vi "Meas Proc QWTB Update Result View Process.vi"(8 "error in":errorcluster, 11 "session in":variant) -> (0 "error out":errorcluster, 3 "QWTB result session out":variant)   [LabVIEW 2020]
doc: "QWTB result viewer: This VI is async. process that will look into current measurement folder. It scans for results header file, then it reads list of the available results for current QWTB algorithm. It fills the result selector by the list of available results.\nThen it tries to load the result data to the table. It also loads descriptions of the table rows which are stored into the QWTB result session. Alternatively it can generate graph of the selected quantity. The decision table vs graph update is made automatically based on the 'QWTB view setup'."
uses:
  Meas Proc QWTB Plot Legend.ctl
  Meas Proc QWTB Viewer Asyn Session.ctl
  Meas Session.ctl
  adc/ADC Session.ctl
  drivers/niScope/niScope Session.ctl
  drivers/niScope/niScope Virtual Channel Config.ctl
  drivers/niScope/niScope Virtual Channel Mode.ctl
  drivers/niScope/niScope Virtual Channel Input Z.ctl
  drivers/niScope/niScope Virtual Channel Coupling.ctl
  drivers/niScope/niScope Type.ctl
  drivers/niScope/niScope Digitizing Process Options.ctl
  drivers/niScope/niScope Data Packet.ctl
  drivers/niScope/niScope Trigger Setup.ctl
  <instrlib>/niScope/Controls/niScope trigger coupling.ctl
  <instrlib>/niScope/Controls/niScope trigger slope.ctl
  drivers/niScope/niScope Reference Clock.ctl
  drivers/DMM/3458A Digitizer Session.ctl
  drivers/DMM/3458A Virtual Channel Config.ctl
  drivers/Counter/Counter Session.ctl
  drivers/Counter/Counter Type.ctl
  drivers/AWG/AWG Session.ctl
  drivers/AWG/AWG Type.ctl
  drivers/AWG/CMI Clock Divider v2/CMI ckd2 Session.ctl
  drivers/AWG/CMI Clock Divider v2/CMI ckd2 Source Mode.ctl
  drivers/AWG/CMI Clock Divider v2/CMI ckd2 Divisor Mode.ctl
  drivers/AWG/CMI Sync V3/CMI Sync V3 session.ctl
  drivers/AWG/CMI Sync V3/Configure/CMI Sync V3 Reference Clock Source.ctl
  drivers/AWG/CMI Sync V3/Configure/CMI Sync V3 HV input Range.ctl
  drivers/AWG/CMI Sync V3/Configure/CMI Sync V3 Trigger Input Level.ctl
  drivers/AWG/CMI Sync V3/Configure/CMI Sync V3 Channel 1 Mode.ctl
  drivers/AWG/CMI Sync V3/Configure/CMI Sync V3 Channel Output Levels.ctl
  drivers/AWG/CMI Sync V3/Configure/CMI Sync V3 Channel 2 Mode.ctl
  drivers/AWG/CMI Sync V3/Configure/CMI Sync V3 Channel 3 Mode.ctl
  drivers/AWG/CMI Sync V3/Configure/CMI Sync V3 Channel 1 Divisor Entry Mode.ctl
  adc/ADC Trig Config.ctl
  adc/ADC Trig Mode Source.ctl
  adc/ADC Trig Slope.ctl
  adc/ADC Trig Coupling.ctl
  drivers/AWG/RaS HMF2500/HMF2500 Config.ctl
  drivers/DMM/3458A Sync Mode.ctl
  drivers/DMM/3458A Idn Mode.ctl
  drivers/DMM/3458A Digitizing Low Levels/Configure/Sampling Mode.ctl
  drivers/DMM/3458A Digitizing Process Options.ctl
  drivers/DMM/3458A Data Packet.ctl
  drivers/DMM/3458A Aux Record Data.ctl
  drivers/DMM/3458A Digitizing Low Levels/Configure/Level Setup.ctl
  drivers/DMM/3458A Digitizing Low Levels/Configure/First Sample Trigger.ctl
  drivers/DMM/3458A Aperture Selection Mode.ctl
  drivers/DMM/3458A Multiplexing Config.ctl
  drivers/Fluke 8588A/F8588A Low Pass Filter.ctl
  drivers/Fluke 8588A/F8588A Phase Lock.ctl
  drivers/Fluke 8588A/F8588A Coupling.ctl
  drivers/DMM/3458A Sampling Rate.ctl
  drivers/AWG/AWG Clock Setup Mode.ctl
  drivers/DMM/3458A Sample Rate Mode.ctl
  drivers/dsdll/DSDLL Session.ctl
  drivers/dsdll/dsdll/dsdll_instance.ctl
  drivers/dsdll/dsdll/dsdll_device_record.ctl
  drivers/dsdll/DSDLL Process Config.ctl
  drivers/dsdll/DSDLL Data Packet.ctl
  adc/ADC Type.ctl
  drivers/simulated_adc/SimAdc Config.ctl
  drivers/simulated_adc/SimAdc Channel Cfg.ctl
  adc/ADC On Close Action.ctl
  adc/Multiplexer/MPX Session.ctl
  adc/Multiplexer/MPX Type.ctl
  drivers/Multiplexers/Generic COM/GCOMM Session.ctl
  drivers/Multiplexers/Generic COM/GCOMM Signal.ctl
  drivers/Multiplexers/Generic COM/GCOMM Virtual Channel.ctl
  drivers/Multiplexers/Generic COM/GCOMM Logic State.ctl
  drivers/Multiplexers/Generic COM/QPMX Session.ctl
  drivers/Multiplexers/QPMX/QPMX switch mode.ctl
  drivers/Multiplexers/QPMX/QPMX polarity.ctl
  drivers/Multiplexers/Generic VISA commands/GVISA Mux Session.ctl
  drivers/Multiplexers/Generic VISA commands/GVISA Mux Path Entry.ctl
  drivers/Multiplexers/Generic VISA commands/met_serial_setup.ctl
  drivers/Agilent DSO 90000/Virtual Digitizer/KeDSO session.ctl
  drivers/Agilent DSO 90000/Virtual Digitizer/KeDSO Virtual Channel.ctl
  drivers/Agilent DSO 90000/Virtual Digitizer/KeDSO High Resolution Mode.ctl
  drivers/Agilent DSO 90000/Virtual Digitizer/KeDSO Trigger Setup.ctl
  drivers/Agilent DSO 90000/Virtual Digitizer/KeDSO Trigger Source.ctl
  drivers/Agilent DSO 90000/Public/Utility/DSO type.ctl
  drivers/cdaq/cDAQ Session.ctl
  drivers/cdaq/low_level_old/cdaq_anal_adc_command.ctl
  drivers/cdaq/low_level_old/cdaq_anal_adc_data.ctl
  drivers/cdaq/cDAQ Virtual Channel.ctl
  drivers/cdaq/cDAQ Master Clock Mode.ctl
  drivers/CMI_ADS127L21/CMI ADS127L21 - Session.ctl
  drivers/CMI_ADS127L21/CMI ADS127L21 - Record Channel.ctl
  drivers/CMI_ADS127L21/CMI ADS127L21 - Input Range.ctl
  drivers/CMI_ADS127L21/CMI ADS127L21 - Input Mode.ctl
  drivers/CMI_ADS127L21/CMI ADS127L21 - Input Impedance.ctl
  drivers/CMI_ADS127L21/CMI ADS127L21 - EXTOUT Mode.ctl
  drivers/CMI_ADS127L21/CMI ADS127L21 - EXTOUT Polarity.ctl
  Meas Sequence Item.ctl
  Meas Sampling Configuration.ctl
  Meas Proc QWTB Algorithm Parameter Data.ctl
  Meas Sequence Configuration.ctl
  Meas Range Mode.ctl
  Meas Sampling Rate Mode.ctl
  octave/golpi/mpc/golpi_session_ref.ctl
  Meas Process Config.ctl
  Meas Process Mode.ctl
  Meas Process Raw Config.ctl
  Meas Process Raw Result Mode.ctl
  Meas Proc QWTB Setup.ctl
  Meas Proc QWTB Uncertainty Mode.ctl
  Meas Proc QWTB Multicore Setup.ctl
  Meas Proc QWTB Multicore Type.ctl
  Meas Process Time Stamp Mode.ctl
  Meas Proc QWTB Exec Mode.ctl
  Corrections/Corr Setup.ctl
  Corrections/Corr Tranducer Item.ctl
  Corrections/Corr Digitizers.ctl
  Assist/Assist Panel Setup.ctl
  Meas Proc QWTB Viewer References.ctl
  Meas Proc QWTB Update Flags.ctl
  Meas Proc QWTB Plot Config.ctl
  Meas Proc QWTB Plot Scale Mode.ctl
  <vilib>/Utility/miscctls.llb/LVRowAndColumnUnsignedTypeDef.ctl
  varilib/SGUI Assign Multiple Strings With Tags By Label.vi
  octave/infolib/1D String.vi
  octave/infolib/Get 1D String.vi
  octave/golpi/Get String.vi
  octave/golpi/Get Double.vi
  octave/golpi/Get 1D Array Double.vi
  octave/golpi/Get 2D Array Double.vi
  octave/golpi/mpc/GOLPI Multi Process.lvlib
  octave/golpi/GOLPI library.lvlib
  varilib/varilib.lvlib
  drivers/niScope/niScope Virtual Digitizer.lvlib
  drivers/DMM/3458A Virtual Digitizer.lvlib
  drivers/Counter/Counter.lvlib
  drivers/AWG/AWG.lvlib
  drivers/DMM/3458A Digitizing Low Levels/3458A Digitizing Low Levels.lvlib
  drivers/dsdll/DSDLL Virtual Digitizer.lvlib
  octave/infolib/infolib.lvlib
  drivers/dsdll/dsdll/dsdll.lvlib
  drivers/AWG/CMI Sync V3/CMI Sync Unit V3.lvlib
  drivers/Agilent DSO 90000/Agilent 90000 Series.lvlib
panel:
  out "user session (memory)":path
  in  "Show legend":T1
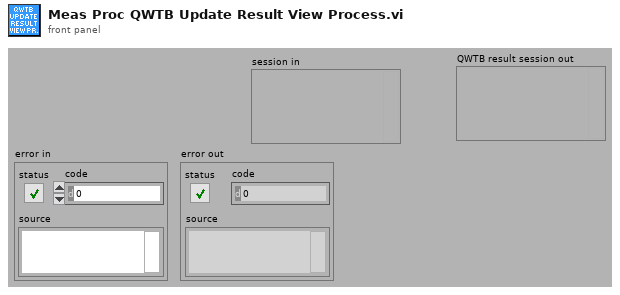
[diagram p1: front panel]
types:
  T1 = typedef "Meas Proc QWTB Plot Legend.ctl" = enum16{"None", "Best", "North", "South", "East", "West", "NorthEast", "NorthWest", "SouthEast", "SouthWest"}
  T2 = typedef "Meas Proc QWTB Viewer Asyn Session.ctl" = cluster{"session":T3, "QWTB result refs":T112, "view setup":T113}
  T3 = typedef "Meas Session.ctl" = cluster{"adc":T4, "sequence":T91[], "sequence setup":T94, "golpi":T97, "processing setup":T98, "corrections":T108, "assist cfg":T111}
  T4 = typedef "ADC Session.ctl" = cluster{"niScope":T5, "3458A":T16, "dsdll":T55, "type":T59, "channel idn str":string[], "aux instr idn str":string[], "modified?":bool, "simadc":T60, "force rst?":bool, "exit mode":T62, "exit dly":dbl, "exit tmr":timestamp, "busy?":bool, "accessed?":bool, "multiplex":T63, "keysight dso":T75, "cdaq":T81, "ignore overload":bool, "ADS127L21":T84}
  T5 = typedef "niScope Virtual Digitizer.lvlib/niScope Session.ctl" = cluster{"channel cfg":T6[], "sessions":refnum<k20>[], "multi cards":bool, "channels":i32, "type":T10, "memory [B/chn]":i32, "ext. clock [Hz]":dbl, "samples count":i64, "use streaming":bool, "proc setup":T11, "sample width [B]":i32, "ranges [V]":dbl[], "trigger setup":T12, "fs [Hz]":dbl, "bitres [bit]":i32, "clock source":T15}
  T6 = typedef "niScope Virtual Digitizer.lvlib/niScope Virtual Channel Config.ctl" = cluster{"Address":refnum<k15>, "Channel":i32, "Mode":T7, "Input Z":T8, "Coupling":T9, "Range [Vpk]":dbl, "btn clr":bool, "btn up":bool, "btn down":bool}
  T7 = typedef "niScope Virtual Digitizer.lvlib/niScope Virtual Channel Mode.ctl" = enum16{"Single ended", "Unbal. differential", "Differential"}
  T8 = typedef "niScope Virtual Digitizer.lvlib/niScope Virtual Channel Input Z.ctl" = enum16{"1 MOhm", "50 Ohm"}
  T9 = typedef "niScope Virtual Digitizer.lvlib/niScope Virtual Channel Coupling.ctl" = enum16{"AC", "DC", "GND"}
  T10 = typedef "niScope Virtual Digitizer.lvlib/niScope Type.ctl" = enum16{"n/a", "5922"}
  T11 = typedef "niScope Virtual Digitizer.lvlib/niScope Digitizing Process Options.ctl" = cluster{"packet size [smpl]":i64, "current timeout [s]":dbl, "blk2blk timeout [s]":dbl, "event time":timestamp, "temp sampl T [s]":dbl, "data queue":refnum<queue>, "stop notifier":refnum<notifier>, "proc ref":refnum<vi>}
  T12 = typedef "niScope Virtual Digitizer.lvlib/niScope Trigger Setup.ctl" = cluster{"coupling":T13, "level [V]":dbl, "slope":T14, "mode":enum16{"Immediate", "External", "Level"}, "pre-trigger [%]":dbl}
  T13 = typedef "niScope trigger coupling.ctl" = u16
  T14 = typedef "niScope trigger slope.ctl" = i32
  T15 = typedef "niScope Virtual Digitizer.lvlib/niScope Reference Clock.ctl" = enum16{"VAL_NO_SOURCE", "VAL_CLK_IN", "VAL_PXI_CLOCK", "VAL_EXTERNAL"}
  T16 = typedef "3458A Virtual Digitizer.lvlib/3458A Digitizer Session.ctl" = cluster{"channels":T17[], "sync unit":T18, "awg unit":T20, "sync mode":T39, "streaming mode":bool, "idn mode":T40, "sampling mode":T41, "sample memory [B]":i32, "proc setup":T42, "sample size [B]":i32, "sample count":i32, "aux data":T44, "ranges [V]":dbl[], "aperture [s]":dbl, "LEVEL trigger":T45, "trigger mode":T46, "measure temp.?":bool, "disp mesages":string[], "shared bus?":bool, "disable display?":bool, "aper mode":T47, "aper rules":dbl[][], "multiplex":T48, "F8588 lpf":T49, "F8588 pll":T50, "F8588 couple":T51, "fs":T52, "fs mode":T54, "init timestamp":timestamp, "last report timestamp":timestamp}
  T17 = typedef "3458A Virtual Digitizer.lvlib/3458A Virtual Channel Config.ctl" = cluster{"VISA":refnum<visa-resource-name>, "Range [Vpk]":dbl, "btn clr":bool, "btn up":bool, "btn down":bool, "F8588":bool, "F8588 guard":bool}
  T18 = typedef "Counter.lvlib/Counter Session.ctl" = cluster{"VISA":refnum<visa-resource-name>, "type":T19}
  T19 = typedef "Counter.lvlib/Counter Type.ctl" = enum16{"Picotest U6200A", "dummy"}
  T20 = typedef "AWG.lvlib/AWG Session.ctl" = cluster{"type":T21, "VISA":refnum<visa-resource-name>, "enable 10MHz ref":bool, "cmi ckd2":T22, "cmi sync v3":T25, "trigger":T34, "HMF2500 cfg":T38}
  T21 = typedef "AWG.lvlib/AWG Type.ctl" = enum16{"Agilent 331xxA to 332xxA", "Agilent 335xxA to 336xxA", "Tektronix AFG3101C", "R&S HMF25xx", "CMI Clock Divider v2", "CMI Sync Unit V3", "dummy"}
  T22 = typedef "AWG.lvlib/CMI ckd2 Session.ctl" = cluster{"VISA":refnum<visa-resource-name>, "clock source":T23, "manual ref clk":bool, "ref clock [Hz]":dbl, "div mode":T24}
  T23 = typedef "AWG.lvlib/CMI ckd2 Source Mode.ctl" = enum16{"Auto", "LF clock", "HF clock", "Internal"}
  T24 = typedef "AWG.lvlib/CMI ckd2 Divisor Mode.ctl" = enum16{"Set divisor directly", "Set divisor by frequency"}
  T25 = typedef "AWG.lvlib/CMI Sync Unit V3.lvlib/CMI Sync V3 session.ctl" = cluster{"VISA":refnum<visa-resource-name>, "baud rate [bd/s]":i32, "source":T26, "hv range":T27, "fsrc is fixed":bool, "fsrc [Hz]":dbl, "freq integ [s]":dbl, "freq filter":i32, "trig level":T28, "chn1 mode":T29, "chn1 level":T30, "chn2 mode":T31, "chn2 level":T30, "chn2 div":i32, "chn3 mode":T32, "chn3 level":T30, "chn1 div entry":T33, "chn1 dev limit [%]":dbl, "chn1 check dev":bool}
  T26 = typedef "AWG.lvlib/CMI Sync Unit V3.lvlib/CMI Sync V3 Reference Clock Source.ctl" = enum16{"Auto", "Internal", "Logic", "Sine", "HV"}
  T27 = typedef "AWG.lvlib/CMI Sync Unit V3.lvlib/CMI Sync V3 HV input Range.ctl" = enum16{"10V", "60V", "250V", "1kV"}
  T28 = typedef "AWG.lvlib/CMI Sync Unit V3.lvlib/CMI Sync V3 Trigger Input Level.ctl" = enum16{"LVCMOS 3V3", "TTL 5V"}
  T29 = typedef "AWG.lvlib/CMI Sync Unit V3.lvlib/CMI Sync V3 Channel 1 Mode.ctl" = enum16{"Source divider", "DDS absolute", "DDS ratio", "DDS ratio M/N"}
  T30 = typedef "AWG.lvlib/CMI Sync Unit V3.lvlib/CMI Sync V3 Channel Output Levels.ctl" = enum16{"Positive 3V3", "Negative 3V3", "Positive 5V", "Negative 5V"}
  T31 = typedef "AWG.lvlib/CMI Sync Unit V3.lvlib/CMI Sync V3 Channel 2 Mode.ctl" = enum16{"Source divider", "Chn 1 divide"}
  T32 = typedef "AWG.lvlib/CMI Sync Unit V3.lvlib/CMI Sync V3 Channel 3 Mode.ctl" = enum16{"Chn 1 Active", "Chn 2 Active", "Chn 1 Trigger", "Chn 2 Trigger", "Gate", "PPS", "10MHz"}
  T33 = typedef "AWG.lvlib/CMI Sync Unit V3.lvlib/CMI Sync V3 Channel 1 Divisor Entry Mode.ctl" = enum16{"Set divisor directly", "Calculate nearest divisor from measured fx"}
  T34 = typedef "ADC Trig Config.ctl" = cluster{"source":T35, "slope":T36, "coupling":T37, "level [V]":dbl, "hysteresis [V]":dbl, "pre-trigger [%]":dbl}
  T35 = typedef "ADC Trig Mode Source.ctl" = enum16{"Immediate", "External", "Level"}
  T36 = typedef "ADC Trig Slope.ctl" = enum16{"POS", "NEG"}
  T37 = typedef "ADC Trig Coupling.ctl" = enum16{"DC", "AC"}
  T38 = typedef "AWG.lvlib/HMF2500 Config.ctl" = cluster{"Baud Rate":u32, "Parity":u16, "Data Bits":u16, "Flow Control":u16}
  T39 = typedef "3458A Virtual Digitizer.lvlib/3458A Sync Mode.ctl" = enum16{"MASTER-SLAVE, MASTER clocked by TIMER", "MASTER-SLAVE, MASTER clocked by AWG", "ALL clocked by AWG", "MASTER-SLAVE, ALL clocked by TIMER", "ALL clocked by AWG with DFLL"}
  T40 = typedef "3458A Virtual Digitizer.lvlib/3458A Idn Mode.ctl" = enum16{"Auto", "Sequential (chn A, chn B, ...)", "From calibration string"}
  T41 = typedef "3458A Virtual Digitizer.lvlib/3458A Digitizing Low Levels.lvlib/Sampling Mode.ctl" = enum16{"DCV", "DSDC", "DSAC"}
  T42 = typedef "3458A Virtual Digitizer.lvlib/3458A Digitizing Process Options.ctl" = cluster{"channel id":i32, "packet size [smpl]":i32, "current timeout [s]":dbl, "blk2blk timeout [s]":dbl, "event time":timestamp, "stop notifier":refnum<notifier>, "data queues":refnum<queue>[], "proc refs":refnum<vi>[], "bus semaphore":T43}
  T43 = typedef "Semaphore RefNum" = refnum<k1>
  T44 = typedef "3458A Virtual Digitizer.lvlib/3458A Aux Record Data.ctl" = cluster{"channel id":i32, "valid?":bool[], "gain [V]":dbl[], "timestamp [s]":dbl[], "Ts [s]":dbl, "abs timestamp":timestamp, "t [deg C]":dbl[], "multiplex timestamp [s]":dbl, "only multiplex?":bool, "multiplex smpl offset":i64, "overflow?":bool}
  T45 = typedef "3458A Virtual Digitizer.lvlib/3458A Digitizing Low Levels.lvlib/Level Setup.ctl" = cluster{"edge":enum16{"POS", "NEG"}, "level [V]":dbl, "coupling":enum16{"DC", "AC"}}
  T46 = typedef "3458A Virtual Digitizer.lvlib/3458A Digitizing Low Levels.lvlib/First Sample Trigger.ctl" = enum16{"AUTO", "EXT", "SYN", "SGL", "HOLD", "LEVEL"}
  T47 = typedef "3458A Virtual Digitizer.lvlib/3458A Aperture Selection Mode.ctl" = enum16{"Manual", "Maximum", "Table"}
  T48 = typedef "3458A Virtual Digitizer.lvlib/3458A Multiplexing Config.ctl" = cluster{"cycles":i32, "delay [s]":dbl, "enabled":bool, "overhead [s]":dbl, "tot smpls":i64, "sub-rec":i32, "overhead [%]":dbl, "emulated":bool}
  T49 = typedef "F8588A Low Pass Filter.ctl" = enum16{"Off", "100 kHz", "3 MHz"}
  T50 = typedef "F8588A Phase Lock.ctl" = enum16{"Off", "1 MHz", "10 MHz"}
  T51 = typedef "F8588A Coupling.ctl" = enum16{"AC, 1 MOhm", "AC, 10 MOhm", "DC, 1 MOhm", "DC, 10 MOhm", "DC, auto"}
  T52 = typedef "3458A Virtual Digitizer.lvlib/3458A Sampling Rate.ctl" = cluster{"freq mode":T53, "fs [Hz]":dbl, "fref [Hz]":dbl, "mul":dbl, "div":dbl}
  T53 = typedef "AWG.lvlib/AWG Clock Setup Mode.ctl" = enum16{"fs or Ts", "fs or Ts with fref", "fref/N", "fref*M/N", "fref*Ratio"}
  T54 = typedef "3458A Sample Rate Mode.ctl" = enum16{"fs or Ts", "fs*M/N"}
  T55 = typedef "DSDLL Virtual Digitizer.lvlib/DSDLL Session.ctl" = cluster{"dsdll":T56, "channels":i32, "device id":i32, "channel idns":string[], "proc setup":T58, "samples count":i32, "fs [Hz]":dbl}
  T56 = typedef "dsdll.lvlib/dsdll_instance.ctl" = cluster{"dsdll path":path, "dsdll handle":u8[], "output devices":T57[], "capture devices":T57[]}
  T57 = typedef "dsdll.lvlib/dsdll_device_record.ctl" = cluster{"guid":u8[], "name":string}
  T58 = typedef "DSDLL Virtual Digitizer.lvlib/DSDLL Process Config.ctl" = cluster{"packet size [smpl]":i32, "current timeout [s]":dbl, "blk2blk timeout [s]":dbl, "event time":timestamp, "data queue":refnum<queue>, "stop notifier":refnum<notifier>, "proc ref":refnum<vi>}
  T59 = typedef "ADC Type.ctl" = enum16{"niScope", "3458A", "DirectSound DLL", "Keysight DSO", "cDAQ ADC", "CMI ADS127L21", "dummy"}
  T60 = typedef "SimAdc Config.ctl" = cluster{"channels":T61[], "range [V]":dbl, "Ts step [s]":dbl, "time [s]":dbl, "fs [Hz]":dbl, "count":i64, "smpl offset":i64, "set count":i64, "bit res":i32}
  T61 = typedef "SimAdc Channel Cfg.ctl" = cluster{"harmonics":dbl[][], "btn clear":bool, "noise":dbl, "fundamental [Hz]":dbl}
  T62 = typedef "ADC On Close Action.ctl" = enum16{"Immediate reset", "Delayed reset"}
  T63 = typedef "MPX Session.ctl" = cluster{"Type":T64, "gen com ssn":T65, "delay before [s]":dbl, "delay post [s]":dbl, "sequence":string[], "enabled":bool, "ref timestamp [s]":dbl, "idn string":string, "dev niScope":refnum<k15>, "niScope idx":i32, "QPMX ssn":T69, "VISA mux ssn":T72}
  T64 = typedef "MPX Type.ctl" = enum16{"Dummy", "Generic - COM port", "Generic - niScope PFI", "Generic - VISA commands", "QPMX"}
  T65 = typedef "GCOMM Session.ctl" = cluster{"visa":refnum<visa-resource-name>, "primary":T66, "secondary":T66, "channels":T67[]}
  T66 = typedef "GCOMM Signal.ctl" = enum16{"None", "DTR", "RTS"}
  T67 = typedef "GCOMM Virtual Channel.ctl" = cluster{"Primary:":T68, "Secondary:":T68, "btn clr":bool, "btn up":bool, "btn down":bool, "Tag:":string}
  T68 = typedef "GCOMM Logic State.ctl" = enum16{"OFF", "ON"}
  T69 = typedef "QPMX Session.ctl" = cluster{"visa":refnum<visa-resource-name>, "switch mode":T70, "sequence":bool[][], "timing delays":u32[], "polarity":T71, "ss delay (s)":dbl, "internal timer (s)":dbl, "Last loaded sequence file":path, "startup delay (s)":dbl}
  T70 = typedef "QPMX switch mode.ctl" = enum16{"Switched by TWM", "Switched by external clock", "Switched by internal clock"}
  T71 = typedef "QPMX polarity.ctl" = enum16{"Positive", "Negative"}
  T72 = typedef "GVISA Mux Session.ctl" = cluster{"VISA":refnum<visa-resource-name>, "paths":T73[], "idn command":string, "serial cfg":T74}
  T73 = typedef "GVISA Mux Path Entry.ctl" = cluster{"Tag:":string, "Command:":string, "btn clr":bool, "btn up":bool, "btn down":bool}
  T74 = typedef "met_serial_setup.ctl" = cluster{"Baud rate":i32, "Data bits":i32, "Parity":i32, "Stop bits":i32, "Flow control":i32, "End Mode Read":enum16{"None", "Last Bit", "TermChar"}, "End Mode Write":enum16{"None", "Last Bit", "TermChar"}, "Term character":u8, "Term enable":bool}
  T75 = typedef "KeDSO session.ctl" = cluster{"VISA":refnum<visa-resource-name>, "channels":T76[], "bw limit [Hz]":dbl, "resolution":T77, "trig noise reject":enum16{"Normal", "High Sensitivity"}, "N":i64, "trigger config":T78, "fs [Hz]":dbl, "timeout stop":timestamp, "waiting for opc":bool, "fetch offset [smpl]":i64, "abs timestamp":timestamp, "ranges [V]":dbl[], "decimation":dbl, "ext ref":bool, "emulate aperture":bool, "model":T80}
  T76 = typedef "KeDSO Virtual Channel.ctl" = cluster{"Channel":i32, "Range [Vpk]":dbl, "btn clr":bool, "btn up":bool, "btn down":bool, "Offset [V]":dbl, "Coupling":enum16{"DC", "DC50", "AC", "LFR1"}, "bw limit enab":bool}
  T77 = typedef "KeDSO High Resolution Mode.ctl" = enum16{"Basic", "High-res AUTO", "Min. 9-bits", "Min. 10-bits", "Min. 11-bits", "Min. 12-bits", "Fixed 11-bits", "Fixed 12-bits", "Fixed 13-bits", "Fixed 14-bits", "Fixed 15-bits", "Fixed 16-bits"}
  T78 = typedef "KeDSO Trigger Setup.ctl" = cluster{"trigger source":T79, "trigger slope":enum16{"Negative", "Positive", "Either"}, "level [V]":dbl, "hysteresis [V]":dbl, "pre-trig [%]":i32}
  T79 = typedef "KeDSO Trigger Source.ctl" = enum16{"Immediate", "Level", "AUX"}
  T80 = typedef "Agilent 90000 Series.lvlib/DSO type.ctl" = enum16{"DSO91304", "DSO91204", "DSO90804", "DSO90604", "DSO90404", "DSO90254", "DSA91304", "DSA91204", "DSA90804", "DSA90604", "DSA90404", "DSA90254", "DSO9104", "DSO9254", "DSO9404", "MSO9104", "MSO9254", "MSO9404", "MSO9064", "DSO9064", "DSOX91604", "DSOX92004", "DSOX92504", "DSOX92804", "DSOX93204", "DSO93004", "DSO9024H", "DSO9054H", "DSO9104H", "DSO9204H", "DSOS054A", "DSOS104A", "DSOS204A", "DSOS254A", "DSOS404A", "DSOS604A", "DSOS804A", "MSOS054A", "MSOS104A", "MSOS204A", "MSOS254A", "MSOS404A", "MSOS604A", "MSOS804A", "DSAX96204Q", "DSOX96204Q", "DSAX95004Q", "DSOX95004Q", "DSAX93304Q", "DSOX93304Q", "DSAX92504Q", "DSOX92504Q", "DSAX92004Q", "DSOX92004Q"}
  T81 = typedef "cDAQ Session.ctl" = cluster{"mclk [Hz]":dbl, "ADC task":refnum<k21>, "mclk reference":string, "fs [Hz]":dbl, "queue adc cmd":refnum<queue>, "queue adc data":refnum<queue>, "adc proc ref":refnum<vi>, "channels":T82[], "last channels":T82[], "timeout":timestamp, "N":i32, "mclk mode":T83, "ext mclk source":tag}
  T82 = typedef "cDAQ Virtual Channel.ctl" = cluster{"Device":tag, "Channel id":i32, "btn clr":bool, "btn up":bool, "btn down":bool}
  T83 = typedef "cDAQ Master Clock Mode.ctl" = enum16{"Free running", "Export master clock", "Import master clock"}
  T84 = typedef "CMI ADS127L21 - Session.ctl" = cluster{"VISA":refnum<visa-resource-name>, "chn list":i32[], "record size":i32, "phys. channels":i32, "adc fifo size":i32, "channels":T85[], "ext refclk?":bool, "fs [Hz]":dbl, "ext refclk [Hz]":dbl, "meas refclk [Hz]":dbl, "EXTOUT mode":T89, "EXTOUT polarity":T90, "EXTOUT divisor":i32}
  T85 = typedef "CMI ADS127L21 - Record Channel.ctl" = cluster{"Range [Vpk]":T86, "Channel":i32, "Mode":T87, "Impedance":T88, "btn clr":bool, "btn up":bool, "btn down":bool}
  T86 = typedef "CMI ADS127L21 - Input Range.ctl" = dbl
  T87 = typedef "CMI ADS127L21 - Input Mode.ctl" = enum16{"Normal", "Inverted", "GND"}
  T88 = typedef "CMI ADS127L21 - Input Impedance.ctl" = enum16{"1M", "1k5"}
  T89 = typedef "CMI ADS127L21 - EXTOUT Mode.ctl" = enum16{"ADCCLK", "REFCLK", "SMPLCLK", "FIRST"}
  T90 = typedef "CMI ADS127L21 - EXTOUT Polarity.ctl" = enum16{"NORM", "INV"}
  T91 = typedef "Meas Sequence Item.ctl" = cluster{"config":T92, "data file path":path, "header file path":path, "group id":i32, "rec id":i32, "group done?":bool, "adc modified?":bool, "source modified?":bool, "progress [%]":dbl, "groups cnt":i32, "rec cnt":i32, "data file relative path":string, "meas root path":path, "calculate?":bool, "comment":string, "avg cnt":i32}
  T92 = typedef "Meas Sampling Configuration.ctl" = cluster{"count [smpl]":i64, "aperture [s]":dbl, "trigger":T34, "ranges [Vpk]":dbl[], "QWTB parameters":T93[], "sampling rate":T52}
  T93 = typedef "Meas Proc QWTB Algorithm Parameter Data.ctl" = cluster{"name":string, "numerics":dbl[], "strings":string[]}
  T94 = typedef "Meas Sequence Configuration.ctl" = cluster{"group setups":T92[], "rec count":i32, "range mode":T95, "fs mode":T96, "rng even":dbl, "rng odd":dbl, "folder":path, "name base":string, "meas id":i32, "settle [s]":dbl, "comment":string, "avg count":i32, "fs-abs-fr fr":dbl, "fs-abs-fr fs":dbl, "fs-div fr":dbl, "fs-div div":dbl, "fs-mn fr":dbl, "fs-mn mul":dbl, "fs-mn div":dbl, "fs-rat fr":dbl, "fs-rat rat":dbl}
  T95 = typedef "Meas Range Mode.ctl" = enum16{"Keep defaults", "Set All channels", "Set Odd and Even channels"}
  T96 = typedef "Meas Sampling Rate Mode.ctl" = enum16{"Frequency", "Period"}
  T97 = typedef "GOLPI Multi Process.lvlib/golpi_session_ref.ctl" = refnum<vi>
  T98 = typedef "Meas Process Config.ctl" = cluster{"mode":T99, "call after avgs?":bool, "calculate?":bool, "raw mode":T100, "QWTB":T102}
  T99 = typedef "Meas Process Mode.ctl" = enum16{"Raw", "QWTB"}
  T100 = typedef "Meas Process Raw Config.ctl" = cluster{"command":string, "result mode":T101, "res variable":string}
  T101 = typedef "Meas Process Raw Result Mode.ctl" = enum16{"Display console output (only Octave)", "Display string variable", "Display result file %respath%"}
  T102 = typedef "Meas Proc QWTB Setup.ctl" = cluster{"QWTB path":path, "alg filter path":string, "alg ids":string[], "alg parameters":string[], "parsed parameters":T93[], "selected alg id":string, "selected unc mode":T103, "qwtb mcc":i32, "qwtb timeout":i32, "qwtb covg":dbl, "qwtb ofs":i64, "qwtb lim data":i64, "multicore":T104, "unc once?":bool, "qwtb tstemp":T106, "octave reset":bool, "exec mode":T107}
  T103 = typedef "Meas Proc QWTB Uncertainty Mode.ctl" = enum16{"None", "GUF", "Monte Carlo"}
  T104 = typedef "Meas Proc QWTB Multicore Setup.ctl" = cluster{"jobs folder":path, "cores":i32, "max jobs":i32, "mode":T105}
  T105 = typedef "Meas Proc QWTB Multicore Type.ctl" = enum16{"Singlecore", "Multicore", "Multistation"}
  T106 = typedef "Meas Process Time Stamp Mode.ctl" = enum16{"Enabled (default)", "Disabled", "Relative to 1. record"}
  T107 = typedef "Meas Proc QWTB Exec Mode.ctl" = enum16{"Single-core", "Parallel Record Processing"}
  T108 = typedef "Corr Setup.ctl" = cluster{"transducers":cluster{"channels":T109[], "last path":path, "root path":path}, "digitizer":T110}
  T109 = typedef "Corr Tranducer Item.ctl" = cluster{"Path":path, "Ratio:":string, "Name:":string, "btn rem":bool, "btn up":bool, "btn down":bool, "s.n.:":string, "btn open":bool, "ratio o/i":dbl, "chn hi":u16, "chn lo":u16, "Phase index":i32, "btn edit":bool, "mpx chn":u16, "btn vdx1":bool, "btn csx1":bool, "invert":bool}
  T110 = typedef "Corr Digitizers.ctl" = cluster{"last path":path, "channel paths":path[], "channel idns":string[], "correction name":string, "channel names":string[], "folders to copy":path[], "channel valid":bool[], "correction path":path, "correction rel path":string, "rel folders to copy":string[], "root path":path}
  T111 = typedef "Assist Panel Setup.ctl" = cluster{"P":i32, "Q":i32, "rel shift":dbl, "ref freq":dbl, "min fs":dbl, "max fs tol":dbl, "min int":dbl, "max int":dbl, "max err":dbl, "max timeout":dbl}
  T112 = typedef "Meas Proc QWTB Viewer References.ctl" = cluster{"tc result":refnum<vi>, "qwtb results tbl":refnum<vi>, "qwtb maxdim":refnum<vi>, "qwtb unc":refnum<vi>, "qwtb order":refnum<vi>, "qwtb maxarr":refnum<vi>, "qwtb res sel":refnum<vi>, "qwtb res info":refnum<vi>, "descriptions":string[], "var names":string[], "channel indexes":i32[], "qwtb ref chn":refnum<vi>, "qwtb ph unit":refnum<vi>, "qwtb alg sel":refnum<vi>, "qwtb meas sel":refnum<vi>, "qwtb ssn info":refnum<vi>, "last session (man)":path, "qwtb qu list":refnum<vi>, "matrix":dbl[][], "comment":string, "qwtb comment":refnum<vi>, "last session":path, "qwtb amp":refnum<vi>}
  T113 = typedef "Meas Proc QWTB Update Flags.ctl" = cluster{"new result":bool, "show graph":bool, "plot setup":T114, "new session":bool, "reset viewer":bool, "store comment":bool}
  T114 = typedef "Meas Proc QWTB Plot Config.ctl" = cluster{"X-axis style":T115, "Y-axis style":T115, "Show legend":T1, "Grid on":bool, "Box on":bool, "show all chn":bool, "keep updating":bool}
  T115 = typedef "Meas Proc QWTB Plot Scale Mode.ctl" = enum16{"Linear", "Log"}
  T116 = typedef "LVRowAndColumnUnsignedTypeDef.ctl" = cluster{"Row":u32, "Column":u32}
  T117 = typedef "GOLPI library.lvlib/GOLPI reference Type Def.ctl" = cluster{"pipe handle":T118, "fast read timeout [ms]":u32, "fast read settle time [ms]":u32, "fast read to multiple [ms]":u32, "max elements per input line":u32, "slow read timeout [ms]":u32, "stdin double format specifier":string, "max elements per stdout output column":u32, "console mode bitstream":bool, "bitstream first read timeout [ms]":u32, "bitstream read timeout [ms]":u32, "struct transfer possible":bool, "matlab mode":bool}
  T118 = typedef "LV Process library.lvlib/Pipe Handle.ctl" = cluster{"lv_proc.dll file path":path, "process instance handle":u32[], "debug mode":bool, "debug data":cluster{"time":timestamp, "stdin":bool, "data":string}[]}
  T119 = typedef "Meas Proc QWTB View Amplitude Mode.ctl" = enum16{"Amplitude", "Effective", "amp. * sqrt(3)", "amp. / sqrt(3)", "eff. * sqrt(3)", "eff. / sqrt(3)", "Peak-Peak", "dB", "dBmV (dBmA)", "dBuV (dBuA)"}
  T120 = typedef "Meas Proc QWTB View Max Dim.ctl" = enum16{"Scalar", "Vector", "Matrix"}
  T121 = typedef "Meas Proc QWTB View Group Mode.ctl" = enum16{"Group quantities", "Group phases"}
  T122 = typedef "Meas Proc QWTB View Uncertainty Mode.ctl" = enum16{"None", "val ± unc", "[val; unc]"}
  T123 = typedef "Meas Proc QWTB View Phase Mode.ctl" = enum16{"± pi [rad]", "0 - 2*pi [rad]", "±180 [deg]", "0 - 360 [deg]"}
  T124 = typedef "LVRowAndColumnTypeDef.ctl" = cluster{"Row":i32, "Column":i32}
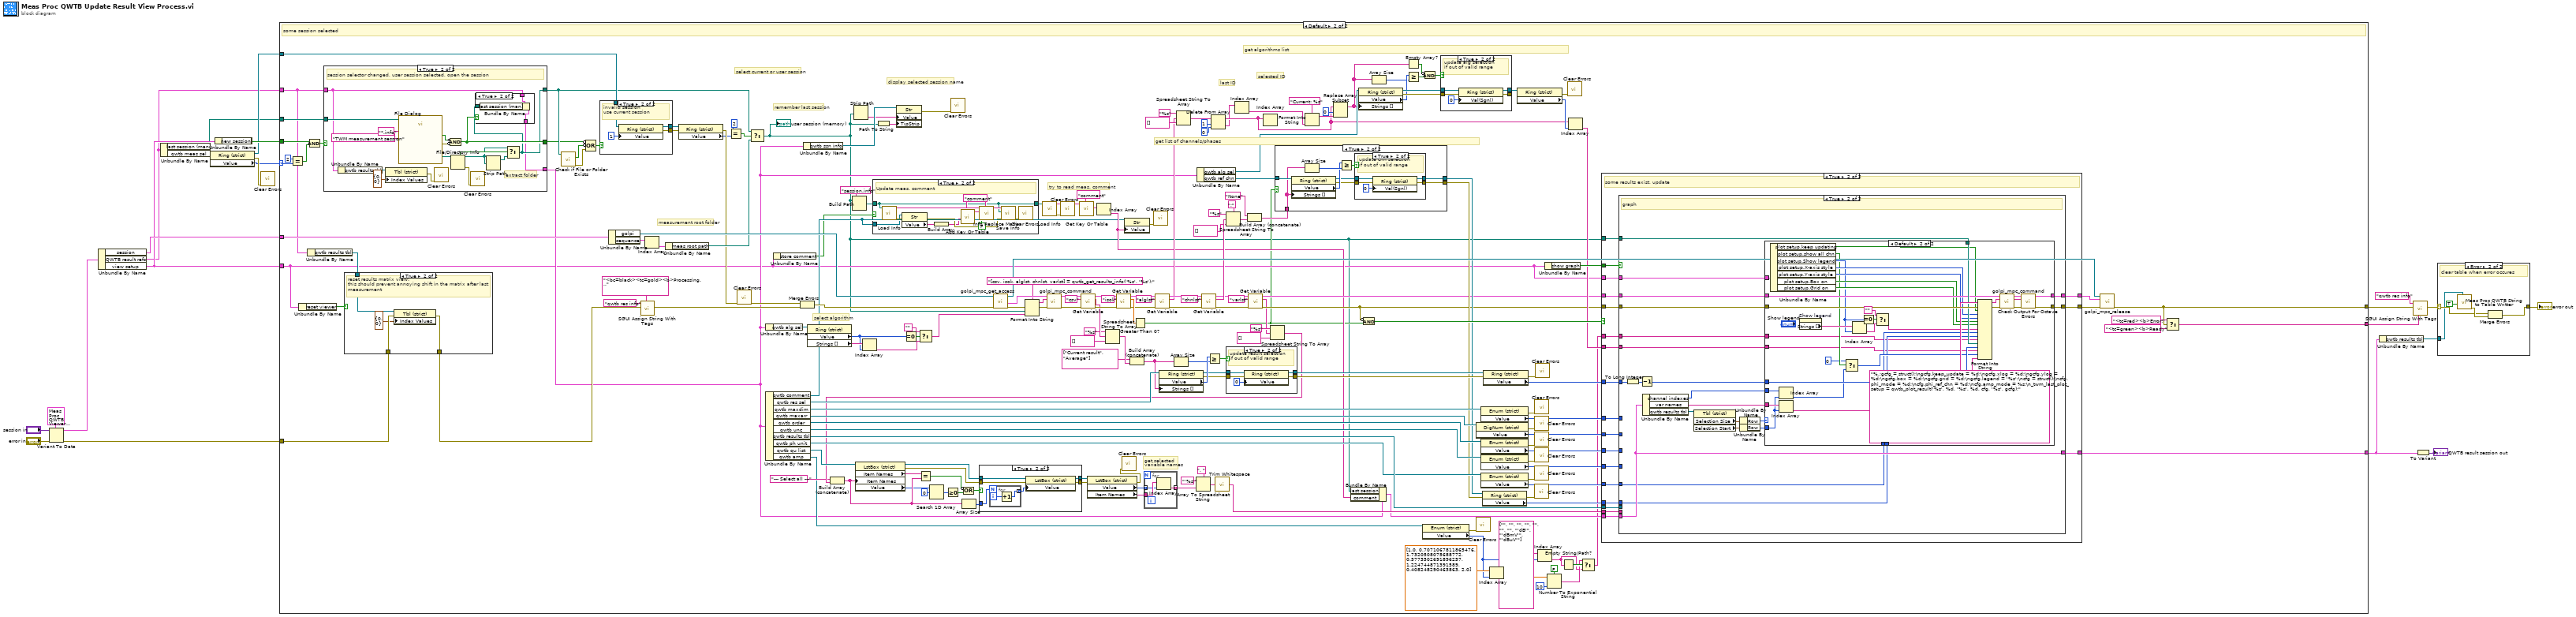
[diagram p0: block diagram]
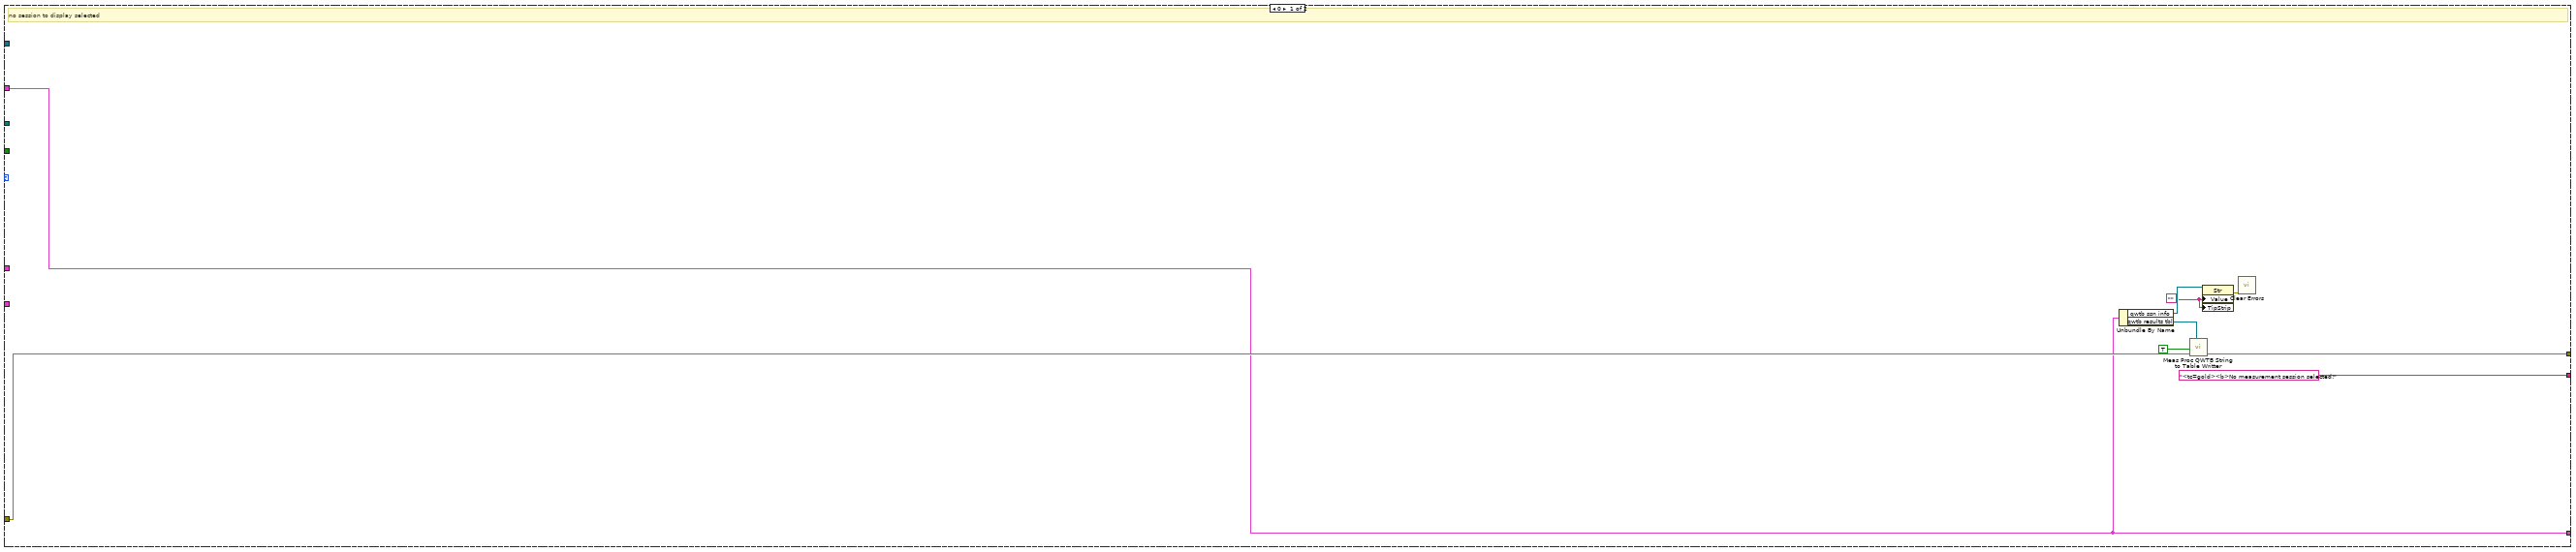
[diagram p3: hidden frame]
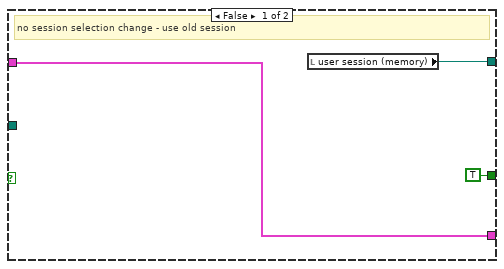
[diagram p10: hidden frame]
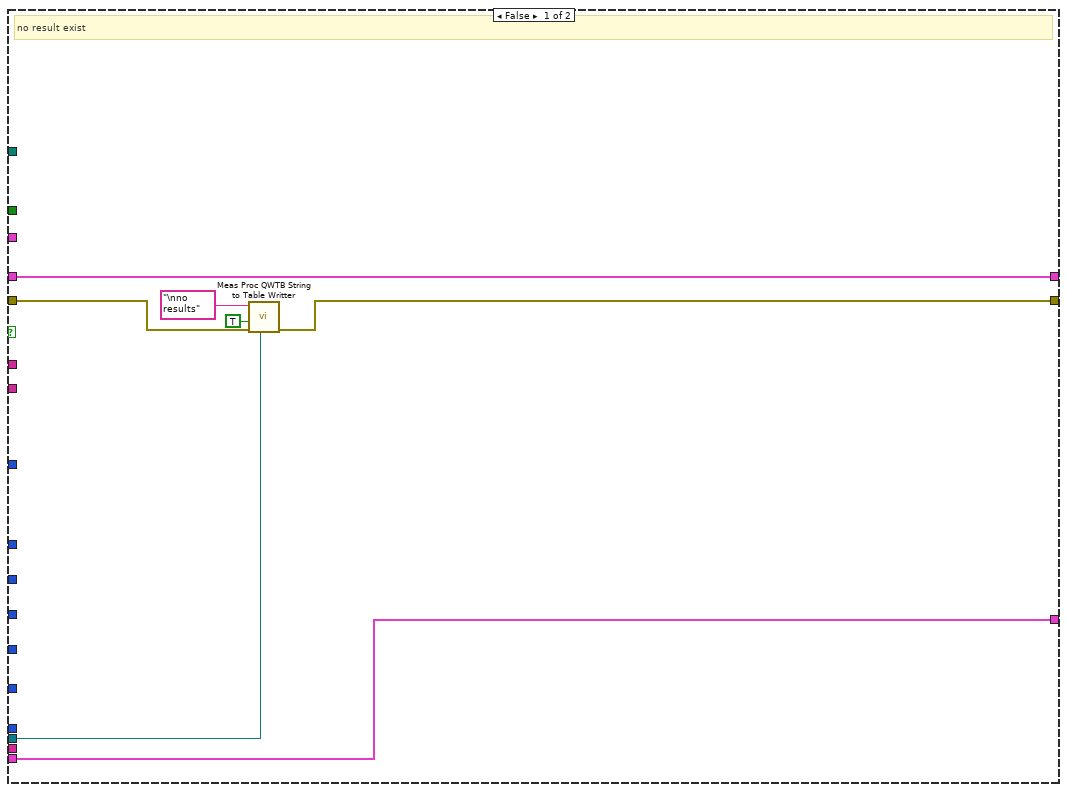
[diagram p13: hidden frame]
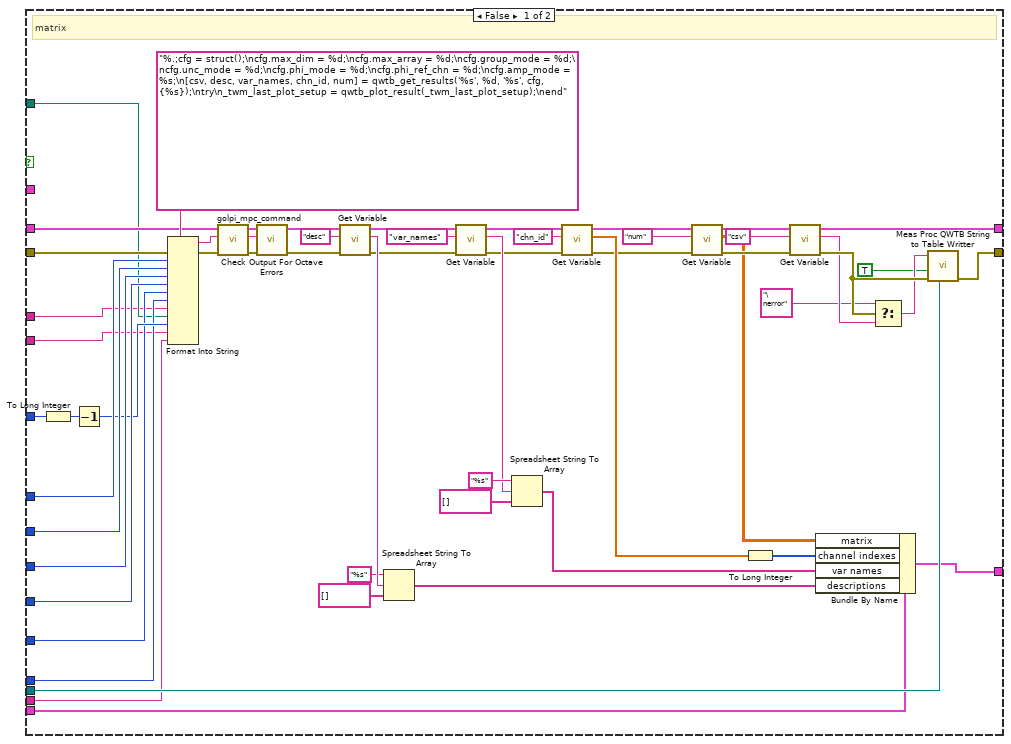
[diagram p14: hidden frame]
diagram:
  n1 = Variant To Data(error in="error in", type=T2 {"session"={"adc"={"niScope"={"channel cfg"=[], "sessions"=[], "multi cards"=FALSE, "channels"=0, "type"=enum."n/a", "memory [B/chn]"=0, "ext. clock [Hz]"=0.0, "samples count"=0, "use streaming"=FALSE, "proc setup"={"packet size [smpl]"=0, "current timeout [s]"=0.0, "blk2blk timeout [s]"=0.0, "event time"=timestamp(0 s since 1904-01-01), "temp sampl T [s]"=0.0, "data queue"=refnum, "stop notifier"=refnum, "proc ref"=refnum}, "sample width [B]"=0, "ranges [V]"=[], "trigger setup"={"coupling"=1, "level [V]"=0.0, "slope"=0, "mode"=enum."Immediate", "pre-trigger [%]"=0.0}, "fs [Hz]"=0.0, "bitres [bit]"=0, "clock source"=enum."VAL_NO_SOURCE"}, "3458A"={"channels"=[], "sync unit"={"VISA"="", "type"=enum."Picotest U6200A"}, "awg unit"={"type"=enum."Agilent 331xxA to 332xxA", "VISA"="", "enable 10MHz ref"=FALSE, "cmi ckd2"={"VISA"="", "clock source"=enum."Auto", "manual ref clk"=FALSE, "ref clock [Hz]"=0.0, "div mode"=enum."Set divisor directly"}, "cmi sync v3"={"VISA"="", "baud rate [bd/s]"=115200, "source"=enum."Auto", "hv range"=enum."1kV", "fsrc is fixed"=FALSE, "fsrc [Hz]"=10000000.0, "freq integ [s]"=1.0, "freq filter"=5, "trig level"=enum."TTL 5V", "chn1 mode"=enum."Source divider", "chn1 level"=enum."Positive 5V", "chn2 mode"=enum."Source divider", "chn2 level"=enum."Positive 5V", "chn2 div"=1, "chn3 mode"=enum."Chn 1 Active", "chn3 level"=enum."Positive 5V", "chn1 div entry"=enum."Calculate nearest divisor from measured fx", "chn1 dev limit [%]"=1.0, "chn1 check dev"=FALSE}, "trigger"={"source"=enum."Immediate", "slope"=enum."POS", "coupling"=enum."DC", "level [V]"=0.0, "hysteresis [V]"=0.0, "pre-trigger [%]"=0.0}, "HMF2500 cfg"={"Baud Rate"=9600, "Parity"=0, "Data Bits"=8, "Flow Control"=4}}, "sync mode"=enum."MASTER-SLAVE, MASTER clocked by TIMER", "streaming mode"=FALSE, "idn mode"=enum."Auto", "sampling mode"=enum."DCV", "sample memory [B]"=0, "proc setup"={"channel id"=0, "packet size [smpl]"=0, "current timeout [s]"=0.0, "blk2blk timeout [s]"=0.0, "event time"=timestamp(0 s since 1904-01-01), "stop notifier"=refnum, "data queues"=[], "proc refs"=[], "bus semaphore"=refnum}, "sample size [B]"=0, "sample count"=0, "aux data"={"channel id"=0, "valid?"=[], "gain [V]"=[], "timestamp [s]"=[], "Ts [s]"=0.0, "abs timestamp"=timestamp(0 s since 1904-01-01), "t [deg C]"=[], "multiplex timestamp [s]"=-1.0, "only multiplex?"=FALSE, "multiplex smpl offset"=0, "overflow?"=FALSE}, "ranges [V]"=[], "aperture [s]"=0.0, "LEVEL trigger"={"edge"=enum."POS", "level [V]"=0.0, "coupling"=enum."DC"}, "trigger mode"=enum."AUTO", "measure temp.?"=FALSE, "disp mesages"=[], "shared bus?"=FALSE, "disable display?"=FALSE, "aper mode"=enum."Manual", "aper rules"=[], "multiplex"={"cycles"=0, "delay [s]"=0.0, "enabled"=FALSE, "overhead [s]"=1.0, "tot smpls"=0, "sub-rec"=0, "overhead [%]"=0.0, "emulated"=FALSE}, "F8588 lpf"=enum."Off", "F8588 pll"=enum."Off", "F8588 couple"=enum."DC, auto", "fs"={"freq mode"=enum."fs or Ts", "fs [Hz]"=0.0, "fref [Hz]"=0.0, "mul"=0.0, "div"=0.0}, "fs mode"=enum."fs or Ts", "init timestamp"=timestamp(0 s since 1904-01-01), "last report timestamp"=timestamp(0 s since 1904-01-01)}, "dsdll"={"dsdll"={"dsdll path"=path "", "dsdll handle"=[], "output devices"=[], "capture devices"=[]}, "channels"=0, "device id"=0, "channel idns"=[], "proc setup"={"packet size [smpl]"=0, "current timeout [s]"=0.0, "blk2blk timeout [s]"=0.0, "event time"=timestamp(0 s since 1904-01-01), "data queue"=refnum, "stop notifier"=refnum, "proc ref"=refnum}, "samples count"=0, "fs [Hz]"=0.0}, "type"=enum."niScope", "channel idn str"=[], "aux instr idn str"=[], "modified?"=FALSE, "simadc"={"channels"=[], "range [V]"=0.0, "Ts step [s]"=0.0, "time [s]"=0.0, "fs [Hz]"=0.0, "count"=0, "smpl offset"=0, "set count"=0, "bit res"=0}, "force rst?"=FALSE, "exit mode"=enum."Immediate reset", "exit dly"=0.0, "exit tmr"=timestamp(0 s since 1904-01-01), "busy?"=FALSE, "accessed?"=FALSE, "multiplex"={"Type"=enum."Dummy", "gen com ssn"={"visa"="", "primary"=enum."None", "secondary"=enum."None", "channels"=[]}, "delay before [s]"=0.0, "delay post [s]"=0.0, "sequence"=[], "enabled"=FALSE, "ref timestamp [s]"=0.0, "idn string"="", "dev niScope"="", "niScope idx"=0, "QPMX ssn"={"visa"="", "switch mode"=enum."Switched by TWM", "sequence"=[], "timing delays"=[], "polarity"=enum."Positive", "ss delay (s)"=2.0, "internal timer (s)"=1.0, "Last loaded sequence file"=path "", "startup delay (s)"=2.0}, "VISA mux ssn"={"VISA"="", "paths"=[], "idn command"="", "serial cfg"={"Baud rate"=9600, "Data bits"=8, "Parity"=0, "Stop bits"=10, "Flow control"=0, "End Mode Read"=enum."None", "End Mode Write"=enum."None", "Term character"=0, "Term enable"=FALSE}}}, "keysight dso"={"VISA"="", "channels"=[], "bw limit [Hz]"=0.0, "resolution"=enum."Basic", "trig noise reject"=enum."Normal", "N"=0, "trigger config"={"trigger source"=enum."Immediate", "trigger slope"=enum."Negative", "level [V]"=0.0, "hysteresis [V]"=0.001, "pre-trig [%]"=50}, "fs [Hz]"=0.0, "timeout stop"=timestamp(0 s since 1904-01-01), "waiting for opc"=FALSE, "fetch offset [smpl]"=0, "abs timestamp"=timestamp(0 s since 1904-01-01), "ranges [V]"=[], "decimation"=1.0, "ext ref"=FALSE, "emulate aperture"=FALSE, "model"=enum."DSO91304"}, "cdaq"={"mclk [Hz]"=12800000.0, "ADC task"="", "mclk reference"="", "fs [Hz]"=50000.0, "queue adc cmd"=refnum, "queue adc data"=refnum, "adc proc ref"=refnum, "channels"=[], "last channels"=[], "timeout"=timestamp(0 s since 1904-01-01), "N"=1000, "mclk mode"=enum."Free running", "ext mclk source"=""}, "ignore overload"=FALSE, "ADS127L21"={"VISA"="", "chn list"=[], "record size"=0, "phys. channels"=0, "adc fifo size"=0, "channels"=[], "ext refclk?"=FALSE, "fs [Hz]"=0.0, "ext refclk [Hz]"=0.0, "meas refclk [Hz]"=0.0, "EXTOUT mode"=enum."ADCCLK", "EXTOUT polarity"=enum."NORM", "EXTOUT divisor"=0}}, "sequence"=[], "sequence setup"={"group setups"=[], "rec count"=0, "range mode"=enum."Keep defaults", "fs mode"=enum."Frequency", "rng even"=0.0, "rng odd"=0.0, "folder"=path "", "name base"="", "meas id"=0, "settle [s]"=0.0, "comment"="", "avg count"=0, "fs-abs-fr fr"=0.0, "fs-abs-fr fs"=0.0, "fs-div fr"=0.0, "fs-div div"=0.0, "fs-mn fr"=0.0, "fs-mn mul"=0.0, "fs-mn div"=0.0, "fs-rat fr"=0.0, "fs-rat rat"=0.0}, "golpi"=refnum, "processing setup"={"mode"=enum."Raw", "call after avgs?"=FALSE, "calculate?"=FALSE, "raw mode"={"command"="", "result mode"=enum."Display console output (only Octave)", "res variable"=""}, "QWTB"={"QWTB path"=path "", "alg filter path"="", "alg ids"=[], "alg parameters"=[], "parsed parameters"=[], "selected alg id"="", "selected unc mode"=enum."None", "qwtb mcc"=100, "qwtb timeout"=90, "qwtb covg"=95.0, "qwtb ofs"=0, "qwtb lim data"=0, "multicore"={"jobs folder"=path "", "cores"=0, "max jobs"=0, "mode"=enum."Singlecore"}, "unc once?"=FALSE, "qwtb tstemp"=enum."Enabled (default)", "octave reset"=FALSE, "exec mode"=enum."Single-core"}}, "corrections"={"transducers"={"channels"=[], "last path"=path "", "root path"=path ""}, "digitizer"={"last path"=path "", "channel paths"=[], "channel idns"=[], "correction name"="", "channel names"=[], "folders to copy"=[], "channel valid"=[], "correction path"=path "", "correction rel path"="", "rel folders to copy"=[], "root path"=path ""}}, "assist cfg"={"P"=0, "Q"=0, "rel shift"=0.0, "ref freq"=0.0, "min fs"=0.0, "max fs tol"=0.0, "min int"=0.0, "max int"=0.0, "max err"=0.0, "max timeout"=0.0}}, "QWTB result refs"={"tc result"=refnum, "qwtb results tbl"=refnum, "qwtb maxdim"=refnum, "qwtb unc"=refnum, "qwtb order"=refnum, "qwtb maxarr"=refnum, "qwtb res sel"=refnum, "qwtb res info"=refnum, "descriptions"=[], "var names"=[], "channel indexes"=[], "qwtb ref chn"=refnum, "qwtb ph unit"=refnum, "qwtb alg sel"=refnum, "qwtb meas sel"=refnum, "qwtb ssn info"=refnum, "last session (man)"=path "", "qwtb qu list"=refnum, "matrix"=[], "comment"="", "qwtb comment"=refnum, "last session"=path "", "qwtb amp"=refnum}, "view setup"={"new result"=FALSE, "show graph"=FALSE, "plot setup"={"X-axis style"=enum."Linear", "Y-axis style"=enum."Linear", "Show legend"=enum."None", "Grid on"=FALSE, "Box on"=FALSE, "show all chn"=FALSE, "keep updating"=FALSE}, "new session"=FALSE, "reset viewer"=FALSE, "store comment"=FALSE}} ("Cluster"), Variant="session in") -> (data=w18:T2, error out=w16:errorcluster)
  n2 = Unbundle By Name(w18) -> ("session"=w17:T3, "QWTB result refs"=w9:T112, "view setup"=w15:T113)
  n3 = Unbundle By Name(w9) -> ("last session (man)"=w10:path, "qwtb meas sel"=w14:refnum<vi>)
  n4 = property class="Ring (strict)"(reference=w14) -> (reference out=w12:refnum<vi>, error out=w11:errorcluster, "Value"=w8:u16)  [unwired: 1 in]
  n5 = Unbundle By Name(w15) -> ("new session"=w13:bool)
  n6 = call <vilib>:"Clear Errors.vi"("error in (no error)"=w11) -> ()  [unwired: 5 in, 2 out]
  n7 = case shown="Default" w8 {
    selector: w8 -> [_ w114]
    tunnel: [w29 w113] -> w6
    tunnel: [w28 w60] -> w2
    tunnel: w17 -> [_ w70]
    tunnel: w16 -> [w30 w67]
    tunnel: w15 -> [_ w51]
    tunnel: w13 -> [_ w139]
    tunnel: w12 -> [_ w135]
    tunnel: w10 -> [_ w124]
    tunnel: w9 -> [w28 w69]
    tunnel: ["<tc=gold><b>No measurement session selected!" ("string (empty)") w112] -> w5
    frame 0 {
      w24 = "" ("Value")
      # "no session to display selected"
      n8 = Unbundle By Name(w28) -> ("qwtb ssn info"=w25:refnum<vi>, "qwtb results tbl"=w27:refnum<vi>)
      n9 = call "Meas Proc QWTB String to Table Writter.vi"("param table ref"=w27, "error in"=w30, "force data update? (False)"=TRUE) -> ("error out"=w29:errorcluster)  [unwired: 7 in, 1 out]
      n10 = property class="Str"(reference=w25, "Value"=w24, "TipStrip"=w24) -> (error out=w23:errorcluster)  [unwired: 1 in, 1 out]
      n11 = call <vilib>:"Clear Errors.vi"("error in (no error)"=w23) -> ()  [unwired: 5 in, 2 out]
    }
    frame Default {
      # "try to read meas. comment"
      # "get selected\nvariable names"
      # "last ID"
      # "selected ID"
      # "display selected session name"
      # "remember last session"
      # "select current or user session"
      # "select algorithm"
      # "get list of channels/phases"
      # "get algorithms list"
      # "measurement root folder"
      # "some session selected"
      n12 = Equal?(x=u16 2, y=w114) -> (x = y?=w118:bool)
      n13 = Unbundle By Name(w51) -> ("reset viewer"=w71:bool)
      n14 = Unbundle By Name(w69) -> ("qwtb results tbl"=w68:refnum<vi>)
      n15 = Compound Arithmetic op=AND(w139, w118) -> (w138:bool)
      n16 = case shown="True" w138 {
        tunnel: [w288 w294] -> w134
        tunnel: [TRUE w295] -> w133
        tunnel: w124 -> [_ w296]
        tunnel: w69 -> [w286 w292]
        tunnel: [w286 w293] -> w59
        frame False {
          # "no session selection change - use old session"
          n17 = local read "user session (memory)"() -> (w288:path)
        }
        frame True {
          # "extract folder"
          # "session selector changed, user session selected, open the session"
          n18 = Unbundle By Name(w292) -> ("qwtb results tbl"=w291:refnum<vi>)
          n19 = property class="Tbl (strict)"(reference=w291, "Index Values"=T116 {"Row"=0, "Column"=0}) -> (error out=w289:errorcluster)  [unwired: 1 in, 1 out]
          n20 = call "File Dialog"("start path"=w296, "pattern (all files)"="*.info", "pattern label"="TWM measurement session") -> ("selected path"=w301:path, "cancelled"=w303:bool, "error out"=w302:errorcluster)  [unwired: 9 in, 1 out]
          n21 = call <vilib>:"Clear Errors.vi"("error in (no error)"=w289) -> ()  [unwired: 5 in, 2 out]
          n22 = Compound Arithmetic op=AND(invert w303, invert w302) -> (w295:bool)
          n23 = File/Directory Info(path=w301) -> (path out=w299:path, directory=w300:bool, error out=w297:errorcluster)  [unwired: 1 in, 4 out]
          n24 = call <vilib>:"Clear Errors.vi"("error in (no error)"=w297) -> ()  [unwired: 5 in, 2 out]
          n25 = Strip Path(path=w299) -> (stripped path=w298:path)  [unwired: 1 out]
          n26 = Select(t=w299, s=w300, f=w298) -> (s? t:f=w294:path)
          n27 = case shown="True" w295 {
            tunnel: w292 -> [w306 w309]
            tunnel: w294 -> [_ w308]
            tunnel: [w306 w307] -> w293
            frame False {
            }
            frame True {
              n28 = Bundle By Name(cluster=w309, "last session (man)"=w308) -> (w307:T112)
            }
          }
        }
      }
      n29 = case shown="True" w71 {
        tunnel: w68 -> [_ w267]
        tunnel: w67 -> [w263 w266]
        tunnel: [w263 w265] -> w66
        frame False {
        }
        frame True {
          # "reset results matrix view:\nthis should prevent annoying shift in the matrix after last \nmeasurement"
          n30 = property class="Tbl (strict)"(reference=w267, error in=w266, "Index Values"=T116 {"Row"=0, "Column"=0}) -> (error out=w265:errorcluster)  [unwired: 1 out]
        }
      }
      n31 = call <vilib>:"Check if File or Folder Exists.vi"("path"=w134) -> ("error out"=w131:errorcluster, "file or folder exists?"=w132:bool)  [unwired: 8 in, 1 out]
      n32 = Compound Arithmetic op=OR(invert w133, invert w132, w131) -> (w130:bool)
      n33 = case shown="True" w130 {
        tunnel: w135 -> [w281 w285]
        tunnel: [w281 w283] -> w136
        tunnel: [_ w282] -> w129
        frame False {
        }
        frame True {
          # "invalid session\nuse current session"
          n34 = property class="Ring (strict)"(reference=w285, "Value"=u16 1) -> (reference out=w283:refnum<vi>, error out=w282:errorcluster)  [unwired: 1 in]
        }
      }
      n35 = Unbundle By Name(w70) -> ("golpi"=w230:T97, "sequence"=w232:T91[])
      n36 = call-poly "SGUI Assign String With Tags.vi"("error in"=w66, "label(s) (empty)"="qwtb res info", "string (empty)"="<bc=black><tc=gold><b>Processing...") -> ("error out"=w123:errorcluster)  [unwired: 7 in, 1 out]
      n37 = Index Array(array=w232) -> (element=w231:T91)  [unwired: 1 in]
      n38 = Unbundle By Name(w231) -> ("meas root path"=w137:path)
      n39 = property class="Ring (strict)"(reference=w136, error in=w129) -> (error out=w128:errorcluster, "Value"=w117:u16)  [unwired: 1 out]
      n40 = Equal?(x=u16 2, y=w117) -> (x = y?=w116:bool)
      n41 = call <vilib>:"Clear Errors.vi"("error in (no error)"=w128) -> ("error out"=w121:errorcluster)  [unwired: 5 in, 1 out]
      n42 = Select(t=w134, s=w116, f=w137) -> (s? t:f=w44:path)
      "user session (memory)" <- w44
      n43 = Unbundle By Name(w59) -> ("qwtb alg sel"=w143:refnum<vi>)
      n44 = Unbundle By Name(w59) -> ("qwtb comment"=w52:refnum<vi>, "qwtb res sel"=w213:refnum<vi>, "qwtb maxdim"=w200:refnum<vi>, "qwtb maxarr"=w199:refnum<vi>, "qwtb order"=w198:refnum<vi>, "qwtb unc"=w197:refnum<vi>, "qwtb results tbl"=w188:refnum<vi>, "qwtb ph unit"=w178:refnum<vi>, "qwtb qu list"=w90:refnum<vi>, "qwtb amp"=w72:refnum<vi>)
      n45 = Unbundle By Name(w51) -> ("store comment"=w50:bool)
      n46 = Merge Errors(w121, w123) -> (w122:errorcluster)
      n47 = Unbundle By Name(w59) -> ("qwtb ssn info"=w127:refnum<vi>)
      n48 = property class="Ring (strict)"(reference=w143) -> ("Value"=w42:u16, "Strings []"=w43:string[])  [unwired: 1 in, 2 out]
      n49 = Build Path(base path=w44, name or relative path="session.info") -> (appended path=w54:path)
      n50 = Strip Path(path=w44) -> (name=w126:string)  [unwired: 1 out]
      n51 = Index Array(array=w43, index=w42) -> (element=w41:string)
      n52 = case shown="True" w50 {
        tunnel: w54 -> [w250 w258]
        tunnel: [w250 w258] -> w53
        tunnel: w52 -> [_ w254]
        frame False {
        }
        frame True {
          w259 = "comment" ("key description to replace")
          # "Update meas. comment"
          n53 = call "Load Info.vi"("filename"=w258) -> ("error out"=w256:errorcluster, "info data"=w262:string)  [unwired: 9 in]
          n54 = property class="Str"(reference=w254, error in=w256) -> (error out=w255:errorcluster, "Value"=w253:string)  [unwired: 1 out]
          n55 = Build Array(w253) -> (w252:string[])
          n56 = call-poly "Add Key Or Table.vi"("key description"=w259, "string"=w252) -> ("info data out"=w260:string)  [unwired: 8 in, 1 out]
          n57 = call "Info Replace Matrix.vi"("key description to replace"=w259, "Allow indent (True)"=FALSE, "info data to paste"=w260, "info data in"=w262) -> ("info data out"=w261:string)  [unwired: 7 in]
          n58 = call "Save Info.vi"("error in"=w255, "filename"=w258, "info data"=w261) -> ("error out"=w257:errorcluster)  [unwired: 8 in]
          n59 = call <vilib>:"Clear Errors.vi"("error in (no error)"=w257) -> ()  [unwired: 5 in, 2 out]
        }
      }
      n60 = Path To String(path=w44) -> (string=w120:string)
      n61 = property class="Str"(reference=w127, "Value"=w126, "TipStrip"=w120) -> (error out=w125:errorcluster)  [unwired: 1 in, 1 out]
      n62 = Equal To 0?(x=w42) -> (x = 0?=w142:bool)
      n63 = Select(t="", s=w142, f=w41) -> (s? t:f=w140:string)
      n64 = call <vilib>:"Clear Errors.vi"("error in (no error)"=w125) -> ()  [unwired: 5 in, 2 out]
      n65 = call "golpi_mpc_get_access.vi"("error in"=w122, "golpi session ref"=w230) -> ("error out"=w228:errorcluster, "GOLPI ref out"=w229:T117, "golpi session ref out (copy)"=w185:T97)  [unwired: 4 in, 3 out]
      n66 = Format Into String(format string="[csv, isok, alglst, chnlst, varlst] = qwtb_get_results_info('%s', '%s');", error in=w228, w44, w140) -> (resulting string=w226:string, error out=w227:errorcluster)  [unwired: 1 in]
      n67 = call "Load Info.vi"("filename"=w53) -> ("error out"=w61:errorcluster, "info data"=w64:string)  [unwired: 9 in]
      n68 = call "golpi_mpc_command.vi"("error in"=w227, "command"=w226, "GOLPI ref in"=w229) -> ("error out"=w224:errorcluster, "GOLPI ref. out"=w223:T117)  [unwired: 6 in, 1 out]
      n69 = call <vilib>:"Clear Errors.vi"("error in (no error)"=w61) -> ()  [unwired: 5 in, 2 out]
      n70 = call-poly "Get Key Or Table.vi"("key description"="comment", "info data"=w64) -> ("value"=w62:string[])  [unwired: 6 in, 3 out]
      n71 = call-poly "Get Variable.vi"("error in"=w224, "variable name"="csv", "GOLPI ref. in"=w223) -> ("error out"=w221:errorcluster, "value"=w217:string, "GOLPI ref. out"=w219:T117)  [unwired: 6 in]
      n72 = Index Array(array=w62) -> (element=w57:string)  [unwired: 1 in]
      n73 = Spreadsheet String To Array(format string="%s", spreadsheet string=w217, array type (2D Dbl)=string[] []) -> (array=w215:string[])  [unwired: 1 in]
      n74 = call-poly "Get Variable.vi"("error in"=w221, "variable name"="isok", "GOLPI ref. in"=w219) -> ("error out"=w163:errorcluster, "value"=w205:dbl, "GOLPI ref. out"=w160:T117)  [unwired: 6 in]
      n75 = property class="Str"(reference=w52, "Value"=w57) -> (error out=w56:errorcluster)  [unwired: 1 in, 1 out]
      n76 = Build Array (concatenate)(string[] ["Current result", "Average"], w215) -> (w212:string[])
      n77 = Greater Than 0?(x=w205) -> (x > 0?=w45:bool)
      n78 = call <vilib>:"Clear Errors.vi"("error in (no error)"=w56) -> ()  [unwired: 5 in, 2 out]
      n79 = call-poly "Get Variable.vi"("error in"=w163, "variable name"="alglst", "GOLPI ref. in"=w160) -> ("error out"=w162:errorcluster, "value"=w156:string, "GOLPI ref. out"=w161:T117)  [unwired: 6 in]
      n80 = property class="Ring (strict)"(reference=w213, "Strings []"=w212) -> (reference out=w208:refnum<vi>, error out=w207:errorcluster, "Value"=w211:u16)  [unwired: 1 in]
      n81 = Array Size(array=w212) -> (size(s)=w210:i32)
      n82 = Spreadsheet String To Array(format string="%s", spreadsheet string=w156, array type (2D Dbl)=string[] []) -> (array=w111:string[])  [unwired: 1 in]
      n83 = Unbundle By Name(w59) -> ("qwtb alg sel"=w148:refnum<vi>, "qwtb ref chn"=w169:refnum<vi>)
      n84 = call-poly "Get Variable.vi"("error in"=w162, "variable name"="chnlst", "GOLPI ref. in"=w161) -> ("error out"=w98:errorcluster, "value"=w173:string, "GOLPI ref. out"=w96:T117)  [unwired: 6 in]
      n85 = Greater Or Equal?(x=w211, y=w210) -> (x >= y?=w209:bool)
      n86 = Delete From Array(array=w111, length=1, index=0) -> (deleted portion=w108:string[], array with subset deleted=w110:string[])
      n87 = Spreadsheet String To Array(delimiter (Tab)=";", format string="%s", spreadsheet string=w173, array type (2D Dbl)=string[] []) -> (array=w168:string[])
      n88 = case shown="True" w209 {
        tunnel: w208 -> [w458 w464]
        tunnel: w207 -> [w459 w463]
        tunnel: [w459 w461] -> w204
        tunnel: [w458 w460] -> w203
        frame False {
        }
        frame True {
          # "update result selection\nif out of valid range"
          n89 = property class="Ring (strict)"(reference=w464, error in=w463, "Value"=u16 0) -> (reference out=w460:refnum<vi>, error out=w461:errorcluster)
        }
      }
      n90 = Index Array(array=w108) -> (element=w107:string)  [unwired: 1 in]
      n91 = Build Array (concatenate)("None" ("delimiter (Tab)"), w168) -> (w166:string[])
      n92 = call-poly "Get Variable.vi"("error in"=w98, "variable name"="varlst", "GOLPI ref. in"=w96) -> ("error out"=w97:errorcluster, "value"=w91:string, "GOLPI ref. out"=w95:T117)  [unwired: 6 in]
      n93 = Index Array(array=w110) -> ()  [unwired: 1 in, 1 out]
      n94 = Spreadsheet String To Array(format string="%s", spreadsheet string=w91, array type (2D Dbl)=string[] []) -> (array=w81:string[])  [unwired: 1 in]
      n95 = Build Array (concatenate)("--- Select all ---", w81) -> (w88:string[])
      n96 = property class="LstBox (strict)"(reference=w90, "Item Names"=w88) -> (reference out=w82:refnum<vi>, error out=w83:errorcluster, "Item Names"=w89:string[], "Value"=w74:i32[])  [unwired: 1 in]
      n97 = Equal?(x=w89, y=w88) -> (x = y?=w85:bool)
      n98 = Search 1D Array(1D array=w74, element=0) -> (index of element=w87:i32)  [unwired: 1 in]
      n99 = Greater Or Equal To 0?(x=w87) -> (x >= 0?=w86:bool)
      n100 = Array Size(array=w88) -> (size(s)=w104:i32)
      n101 = Compound Arithmetic op=OR(invert w85, w86) -> (w84:bool)
      n102 = case shown="True" w84 {
        tunnel: w82 -> [w272 w278]
        tunnel: w104 -> [_ w277]
        tunnel: [w272 w276] -> w103
        tunnel: w83 -> [w271 w275]
        tunnel: [w271 w274] -> w100
        frame False {
        }
        frame True {
          n103 = for {
            N: w277 -> [_]
            tunnel: [w279] -> w273 mode=indexing
            i -> [w280]
            n104 = Increment(x=w280) -> (x+1=w279:i32)
          }
          n105 = property class="LstBox (strict)"(reference=w278, error in=w275, "Value"=w273) -> (reference out=w276:refnum<vi>, error out=w274:errorcluster)
        }
      }
      n106 = property class="LstBox (strict)"(reference=w103, error in=w100) -> (error out=w99:errorcluster, "Value"=w102:i32[], "Item Names"=w101:string[])  [unwired: 1 out]
      n107 = call <vilib>:"Clear Errors.vi"("error in (no error)"=w99) -> ()  [unwired: 5 in, 2 out]
      n108 = for {
        tunnel: w102 -> [w269] mode=indexing
        tunnel: w101 -> [w270]
        tunnel: [w268] -> w79 mode=indexing
        n109 = Index Array(array=w270, index=w269) -> (element=w268:string)
      }
      n110 = Array To Spreadsheet String(delimiter (Tab)=", ", array=w79, 3:"'%s'" ("format string")) -> (spreadsheet string=w76:string)
      n111 = call <vilib>:"Trim Whitespace.vi"("string"=w76) -> ("trimmed string"=w75:string)  [unwired: 1 in]
      n112 = case shown="True" w45 {
        tunnel: w169 -> [w233 w242]
        tunnel: w166 -> [_ w241]
        tunnel: [w233 w235] -> w165
        tunnel: [_ w234] -> w164
        frame False {
        }
        frame True {
          n113 = property class="Ring (strict)"(reference=w242, "Strings []"=w241) -> (reference out=w237:refnum<vi>, error out=w236:errorcluster, "Value"=w239:u16)  [unwired: 1 in]
          n114 = Array Size(array=w241) -> (size(s)=w240:i32)
          n115 = Greater Or Equal?(x=w239, y=w240) -> (x >= y?=w238:bool)
          n116 = case shown="True" w238 {
            tunnel: w237 -> [w243 w249]
            tunnel: w236 -> [w244 w248]
            tunnel: [w244 w246] -> w234
            tunnel: [w243 w245] -> w235
            frame False {
            }
            frame True {
              # "update chn selection\nif out of valid range"
              n117 = property class="Ring (strict)"(reference=w249, error in=w248, "Val(Sgnl)"=u16 0 ("Value")) -> (reference out=w245:refnum<vi>, error out=w246:errorcluster)
            }
          }
        }
      }
      n118 = Format Into String(format string="Current: %s" ("delimiter (Tab)"), w107) -> (resulting string=w154:string)  [unwired: 2 in, 1 out]
      n119 = Replace Array Subset(array=w110, new element=w154, index=0) -> (w46:string[])
      n120 = Bundle By Name(cluster=w59, "last session"=w44, "comment"=w57) -> (w58:T112)
      n121 = property class="Ring (strict)"(reference=w148, "Strings []"=w46) -> (reference out=w151:refnum<vi>, error out=w152:errorcluster, "Value"=w150:u16)  [unwired: 1 in]
      n122 = Compound Arithmetic op=AND(invert w97, w45) -> (w206:bool)
      n123 = Array Size(array=w46) -> (size(s)=w149:i32)
      n124 = Empty Array?(array=w46) -> (empty?=w47:bool)
      n125 = Greater Or Equal?(x=w150, y=w149) -> (x >= y?=w49:bool)
      n126 = property class="Enum (strict)"(reference=w72) -> (error out=w73:errorcluster, "Value"=w39:T119)  [unwired: 1 in, 1 out]
      n127 = Compound Arithmetic op=AND(invert w47, w49) -> (w48:bool)
      n128 = case shown="True" w48 {
        tunnel: w151 -> [w310 w316]
        tunnel: w152 -> [w311 w315]
        tunnel: [w311 w313] -> _
        tunnel: [w310 w312] -> w147
        frame False {
        }
        frame True {
          # "update alg selection\nif out of valid range"
          n129 = property class="Ring (strict)"(reference=w316, error in=w315, "Val(Sgnl)"=u16 0 ("Value")) -> (reference out=w312:refnum<vi>, error out=w313:errorcluster)
        }
      }
      n130 = call <vilib>:"Clear Errors.vi"("error in (no error)"=w73) -> ()  [unwired: 5 in, 2 out]
      n131 = property class="DigNum (strict)"(reference=w199) -> (error out=w195:errorcluster, "Value"=w191:i32)  [unwired: 1 in, 1 out]
      n132 = property class="Enum (strict)"(reference=w200) -> (error out=w196:errorcluster, "Value"=w192:T120)  [unwired: 1 in, 1 out]
      n133 = property class="Enum (strict)"(reference=w198) -> (error out=w194:errorcluster, "Value"=w190:T121)  [unwired: 1 in, 1 out]
      n134 = property class="Enum (strict)"(reference=w197) -> (error out=w193:errorcluster, "Value"=w189:T122)  [unwired: 1 in, 1 out]
      n135 = property class="Enum (strict)"(reference=w178) -> (error out=w179:errorcluster, "Value"=w177:T123)  [unwired: 1 in, 1 out]
      n136 = property class="Ring (strict)"(reference=w165, error in=w164) -> (error out=w176:errorcluster, "Value"=w175:u16)  [unwired: 1 out]
      n137 = property class="Ring (strict)"(reference=w203, error in=w204) -> (error out=w202:errorcluster, "Value"=w201:u16)  [unwired: 1 out]
      n138 = Index Array(array=dbl[] [1.0, 0.7071067811865476, 1.7320508075688772, 0.5773502691896257, 1.224744871391589, 0.408248290463863, 2.0], index=w39) -> (element=w38:dbl)
      n139 = property class="Ring (strict)"(reference=w147) -> (error out=w145:errorcluster, "Value"=w146:u16)  [unwired: 1 in, 1 out]
      n140 = call <vilib>:"Clear Errors.vi"("error in (no error)"=w176) -> ()  [unwired: 5 in, 2 out]
      n141 = call <vilib>:"Clear Errors.vi"("error in (no error)"=w196) -> ()  [unwired: 5 in, 2 out]
      n142 = call <vilib>:"Clear Errors.vi"("error in (no error)"=w195) -> ()  [unwired: 5 in, 2 out]
      n143 = call <vilib>:"Clear Errors.vi"("error in (no error)"=w194) -> ()  [unwired: 5 in, 2 out]
      n144 = call <vilib>:"Clear Errors.vi"("error in (no error)"=w193) -> ()  [unwired: 5 in, 2 out]
      n145 = call <vilib>:"Clear Errors.vi"("error in (no error)"=w179) -> ()  [unwired: 5 in, 2 out]
      n146 = call <vilib>:"Clear Errors.vi"("error in (no error)"=w202) -> ()  [unwired: 5 in, 2 out]
      n147 = Index Array(array=string[] ["", "", "", "", "", "", "", "'dB'", "'dBmV'", "'dBuV'"], index=w39) -> (element=w33:string)
      n148 = Unbundle By Name(w51) -> ("show graph"=w180:bool)
      n149 = Number To Exponential String(number=w38, precision (6)=i16 10, 1:FALSE ("use system decimal point (T)")) -> (E-format string=w34:string)  [unwired: 1 in]
      n150 = Empty String/Path?(string/path=w33) -> (empty?=w35:bool)
      n151 = call <vilib>:"Clear Errors.vi"("error in (no error)"=w145) -> ()  [unwired: 5 in, 2 out]
      n152 = Index Array(array=w110, index=w146) -> (element=w144:string)
      n153 = Select(t=w34, s=w35, f=w33) -> (s? t:f=w32:string)
      n154 = case shown="True" w206 {
        tunnel: w201 -> [_ w337]
        tunnel: w97 -> [w323 w343]
        tunnel: w192 -> [_ w342]
        tunnel: w191 -> [_ w341]
        tunnel: w190 -> [_ w340]
        tunnel: w189 -> [_ w339]
        tunnel: w44 -> [_ w338]
        tunnel: w95 -> [w320 w336]
        tunnel: w188 -> [w321 w335]
        tunnel: [w319 w334] -> w187
        tunnel: [w320 w333] -> w186
        tunnel: w58 -> [w317 w332]
        tunnel: [w317 w331] -> w60
        tunnel: w180 -> [_ w330]
        tunnel: w51 -> [_ w329]
        tunnel: w177 -> [_ w328]
        tunnel: w175 -> [_ w327]
        tunnel: w144 -> [_ w326]
        tunnel: w75 -> [_ w325]
        tunnel: w32 -> [_ w324]
        frame False {
          # "no result exist"
          n155 = call "Meas Proc QWTB String to Table Writter.vi"("param table ref"=w321, "error in"=w323, "force data update? (False)"=TRUE, "content csv string"="\nno results" ("control string")) -> ("error out"=w319:errorcluster)  [unwired: 6 in, 1 out]
        }
        frame True {
          # "some results exist, update"
          n156 = case shown="True" w330 {
            tunnel: w343 -> [w397 w420]
            tunnel: w342 -> [w395 _]
            tunnel: w341 -> [w394 _]
            tunnel: w340 -> [w393 _]
            tunnel: w339 -> [w392 _]
            tunnel: w338 -> [w351 w414]
            tunnel: w337 -> [w391 w419]
            tunnel: w336 -> [w390 w418]
            tunnel: w335 -> [w386 _]
            tunnel: [w381 w415] -> w334
            tunnel: [w380 w416] -> w333
            tunnel: w332 -> [w370 w412]
            tunnel: [w368 w412] -> w331
            tunnel: w329 -> [_ w405]
            tunnel: w328 -> [w355 w403]
            tunnel: w327 -> [w354 w402]
            tunnel: w326 -> [w353 w401]
            tunnel: w325 -> [w352 _]
            tunnel: w324 -> [w350 w400]
            frame False {
              # "matrix"
              n157 = To Long Integer(number=w391) -> (32bit integer=w378:i32)
              n158 = Decrement(x=w378) -> (x-1=w379:i32)
              n159 = Format Into String(format string="%.;cfg = struct();\ncfg.max_dim = %d;\ncfg.max_array = %d;\ncfg.group_mode = %d;\ncfg.unc_mode = %d;\ncfg.phi_mode = %d;\ncfg.phi_ref_chn = %d;\ncfg.amp_mode = %s;\n[csv, desc, var_names, chn_id, num] = qwtb_get_results('%s', %d, '%s', cfg, {%s});\ntry\n_twm_last_plot_setup = qwtb_plot_result(_twm_last_plot_setup);\nend", error in=w397, w395, w394, w393, w392, w355, w354, w350, w351, w379, w353, w352) -> (resulting string=w399:string, error out=w398:errorcluster)  [unwired: 1 in]
              n160 = call "golpi_mpc_command.vi"("error in"=w398, "command"=w399, "GOLPI ref in"=w390) -> ("error out"=w387:errorcluster, "read buffer"=w388:string, "GOLPI ref. out"=w374:T117)  [unwired: 6 in]
              n161 = call "Check Output For Octave Errors.vi"("error in"=w387, "read buffer"=w388) -> ("error out"=w375:errorcluster)  [unwired: 9 in]
              n162 = call-poly "Get Variable.vi"("error in"=w375, "variable name"="desc", "GOLPI ref. in"=w374) -> ("error out"=w366:errorcluster, "value"=w373:string, "GOLPI ref. out"=w365:T117)  [unwired: 6 in]
              n163 = Spreadsheet String To Array(format string="%s", spreadsheet string=w373, array type (2D Dbl)=string[] []) -> (array=w369:string[])  [unwired: 1 in]
              n164 = call-poly "Get Variable.vi"("error in"=w366, "variable name"="var_names", "GOLPI ref. in"=w365) -> ("error out"=w360:errorcluster, "value"=w362:string, "GOLPI ref. out"=w359:T117)  [unwired: 6 in]
              n165 = Spreadsheet String To Array(format string="%s", spreadsheet string=w362, array type (2D Dbl)=string[] []) -> (array=w361:string[])  [unwired: 1 in]
              n166 = call-poly "Get Variable.vi"("error in"=w360, "variable name"="chn_id", "GOLPI ref. in"=w359) -> ("error out"=w348:errorcluster, "value"=w357:dbl[], "GOLPI ref. out"=w347:T117)  [unwired: 6 in]
              n167 = call-poly "Get Variable.vi"("error in"=w348, "variable name"="num", "GOLPI ref. in"=w347) -> ("error out"=w346:errorcluster, "value"=w344:dbl[][], "GOLPI ref. out"=w345:T117)  [unwired: 6 in]
              n168 = To Long Integer(number=w357) -> (32bit integer=w356:i32[])
              n169 = call-poly "Get Variable.vi"("error in"=w346, "variable name"="csv", "GOLPI ref. in"=w345) -> ("error out"=w385:errorcluster, "value"=w383:string, "GOLPI ref. out"=w380:T117)  [unwired: 6 in]
              n170 = Bundle By Name(cluster=w370, "matrix"=w344, "channel indexes"=w356, "var names"=w361, "descriptions"=w369) -> (w368:T112)
              n171 = Select(t="\nerror", s=w385, f=w383) -> (s? t:f=w384:string)
              n172 = call "Meas Proc QWTB String to Table Writter.vi"("param table ref"=w386, "error in"=w385, "force data update? (False)"=TRUE, "content csv string"=w384) -> ("error out"=w381:errorcluster)  [unwired: 6 in, 1 out]
            }
            frame True {
              # "graph"
              n173 = To Long Integer(number=w419) -> (32bit integer=w417:i32)
              n174 = Decrement(x=w417) -> (x-1=w413:i32)
              n175 = Unbundle By Name(w412) -> ("channel indexes"=w404:i32[], "var names"=w406:string[], "qwtb results tbl"=w411:refnum<vi>)
              n176 = property class="Tbl (strict)"(reference=w411) -> ("Selection Size"=w410:T124, "Selection Start"=w409:T124)  [unwired: 1 in, 2 out]
              n177 = Unbundle By Name(w410) -> ("Row"=w408:i32)
              n178 = Unbundle By Name(w409) -> ("Row"=w407:i32)
              n179 = case shown="Default" w408 {
                tunnel: w420 -> [w422 w455]
                tunnel: w418 -> [w421 w445]
                tunnel: [w421 w451] -> w416
                tunnel: [w422 w450] -> w415
                tunnel: w414 -> [_ w449]
                tunnel: w413 -> [_ w448]
                tunnel: w407 -> [_ w432]
                tunnel: w406 -> [_ w447]
                tunnel: w405 -> [_ w444]
                tunnel: w404 -> [_ w433]
                tunnel: w403 -> [_ w427]
                tunnel: w402 -> [_ w426]
                tunnel: w401 -> [_ w425]
                tunnel: w400 -> [_ w424]
                frame 0 {
                }
                frame Default {
                  n180 = Unbundle By Name(w444) -> ("plot setup.keep updating"=w423:bool, "plot setup.show all chn"=w431:bool, "plot setup.Show legend"=w438:T1, "plot setup.X-axis style"=w443:T115, "plot setup.Y-axis style"=w442:T115, "plot setup.Box on"=w441:bool, "plot setup.Grid on"=w440:bool)
                  n181 = Index Array(array=w433, index=w432) -> (element=w430:i32)
                  n182 = Index Array(array=w447, index=w432) -> (element=w446:string)
                  n183 = property on="Show legend" class="Enum (strict)"() -> ("Strings []"=w439:string[])  [unwired: 2 in, 2 out]
                  n184 = Select(t=0, s=w431, f=w430) -> (s? t:f=w428:i32)
                  n185 = Index Array(array=w439, index=w438) -> (element=w436:string)
                  n186 = Equal To 0?(x=w438) -> (x = 0?=w437:bool)
                  n187 = Select(t="", s=w437, f=w436) -> (s? t:f=w434:string)
                  n188 = Format Into String(format string="%.;gcfg = struct();\ngcfg.keep_update = %d;\ngcfg.xlog = %d;\ngcfg.ylog = %d;\ngcfg.box = %d;\ngcfg.grid = %d;\ngcfg.legend = '%s';\ncfg = struct();\ncfg.phi_mode = %d;\ncfg.phi_ref_chn = %d;\ncfg.amp_mode = %s;\n_twm_last_plot_setup = qwtb_plot_result('%s', %d, '%s', %d, cfg, '%s', gcfg);", error in=w455, w423, w443, w442, w441, w440, w434, w427, w426, w424, w449, w448, w425, w428, w446) -> (resulting string=w457:string, error out=w456:errorcluster)  [unwired: 1 in]
                  n189 = call "golpi_mpc_command.vi"("error in"=w456, "command"=w457, "GOLPI ref in"=w445) -> ("error out"=w452:errorcluster, "read buffer"=w453:string, "GOLPI ref. out"=w451:T117)  [unwired: 6 in]
                  n190 = call "Check Output For Octave Errors.vi"("error in"=w452, "read buffer"=w453) -> ("error out"=w450:errorcluster)  [unwired: 9 in]
                }
              }
            }
          }
        }
      }
      n191 = call "golpi_mpc_release.vi"("error in"=w187, "golpi ref or golpi session in"=w186, "golpi session ref"=w185) -> ("error out"=w113:errorcluster)  [unwired: 7 in, 1 out]
      n192 = Select(t="<tc=red><b>Error!" ("string (empty)"), s=w113, f="<tc=green><b>Ready" ("string (empty)")) -> (s? t:f=w112:string)
    }
  }
  n193 = Unbundle By Name(w2) -> ("qwtb results tbl"=w1:refnum<vi>)
  n194 = call-poly "SGUI Assign String With Tags.vi"("error in"=w6, "label(s) (empty)"="qwtb res info", "string (empty)"=w5) -> ("error out"=w4:errorcluster)  [unwired: 7 in, 1 out]
  n195 = To Variant(anything=w2) -> (Variant=→"QWTB result session out":variant)
  n196 = case shown="Error" w4 {
    selector: w4 -> [w465 w469]
    tunnel: [w465 w468] -> w3
    tunnel: w1 -> [_ w467]
    frame No Error {
    }
    frame Error {
      # "clear table when error occures"
      n197 = call "Meas Proc QWTB String to Table Writter.vi"("param table ref"=w467, "force data update? (False)"=TRUE) -> ("error out"=w470:errorcluster)  [unwired: 8 in, 1 out]
      n198 = Merge Errors(w469, w470) -> (w468:errorcluster)
    }
  }
  "error out" <- w3
